vi "Converter_1.0.2_to_1.0.3.vi"() -> ()   [LabVIEW 2014]
uses:
  <vilib>/Utility/xml.llb/Read From XML File(string).vi
panel:
  out "Datenspeicher 2":T1={"Fahrzeugdaten"="", "date/time string"="", "Rolle [Inkr/U]"=0, "Rollenumfang [m]"=0.0, "Rollenträgheit [kgm²]"=0.0, "Zündung [Imp/U]"=0, "Getriebe [1:]"=0.0, "Reifenumfang [m] "=0.0, "element"=0.0, "Gl. Mittelwert"=0, "Differenzenquotient"=0, "Polynom"=0, "element"=0.0, "element"=0.0, "Lufttemperatur [°C]"=0.0, "Luftfeuchtigkeit [%]"=0.0, "Luftdruck [mbar]"=0.0, [], [], "Best Polynomial Fit"=[], [], "Übersetzung ermitteln aus"=0, "[s]"=0.0, "nmin [1/min]"=0.0, "nmax [1/min]"=0.0, "n vom Gas [1/min]"=0.0, [], [], "Boolesch"=FALSE, "Serielle Schnittstelle"="COM4"}
  out "Datenspeicher":T2={"Fahrzeugdaten"="", "date/time string"="", "Rolle [Inkr/U]"=0, "Rollenumfang [m]"=0.0, "Rollenträgheit [kgm²]"=0.0, "Zündung [Imp/U]"=0.0, "Getriebe [1:]"=0.0, "Reifenumfang [m] "=0.0, "element"=0.0, "Gl. Mittelwert"=0, "Differenzenquotient"=0, "Polynom"=0, "element"=0.0, "element"=0.0, "Lufttemperatur [°C]"=0.0, "Luftfeuchtigkeit [%]"=0.0, "Luftdruck [mbar]"=0.0, [], [], "Best Polynomial Fit"=[], [], "Übersetzung ermitteln aus"=0, "[s]"=0.0, "nmin [1/min]"=0.0, "nmax [1/min]"=0.0, "n vom Gas [1/min]"=0.0, [], [], "Boolesch"=FALSE, "Serielle Schnittstelle"="COM4", "nKuWe/nRolle"=10.0}
  # "WildBugChilGru XML Converter"
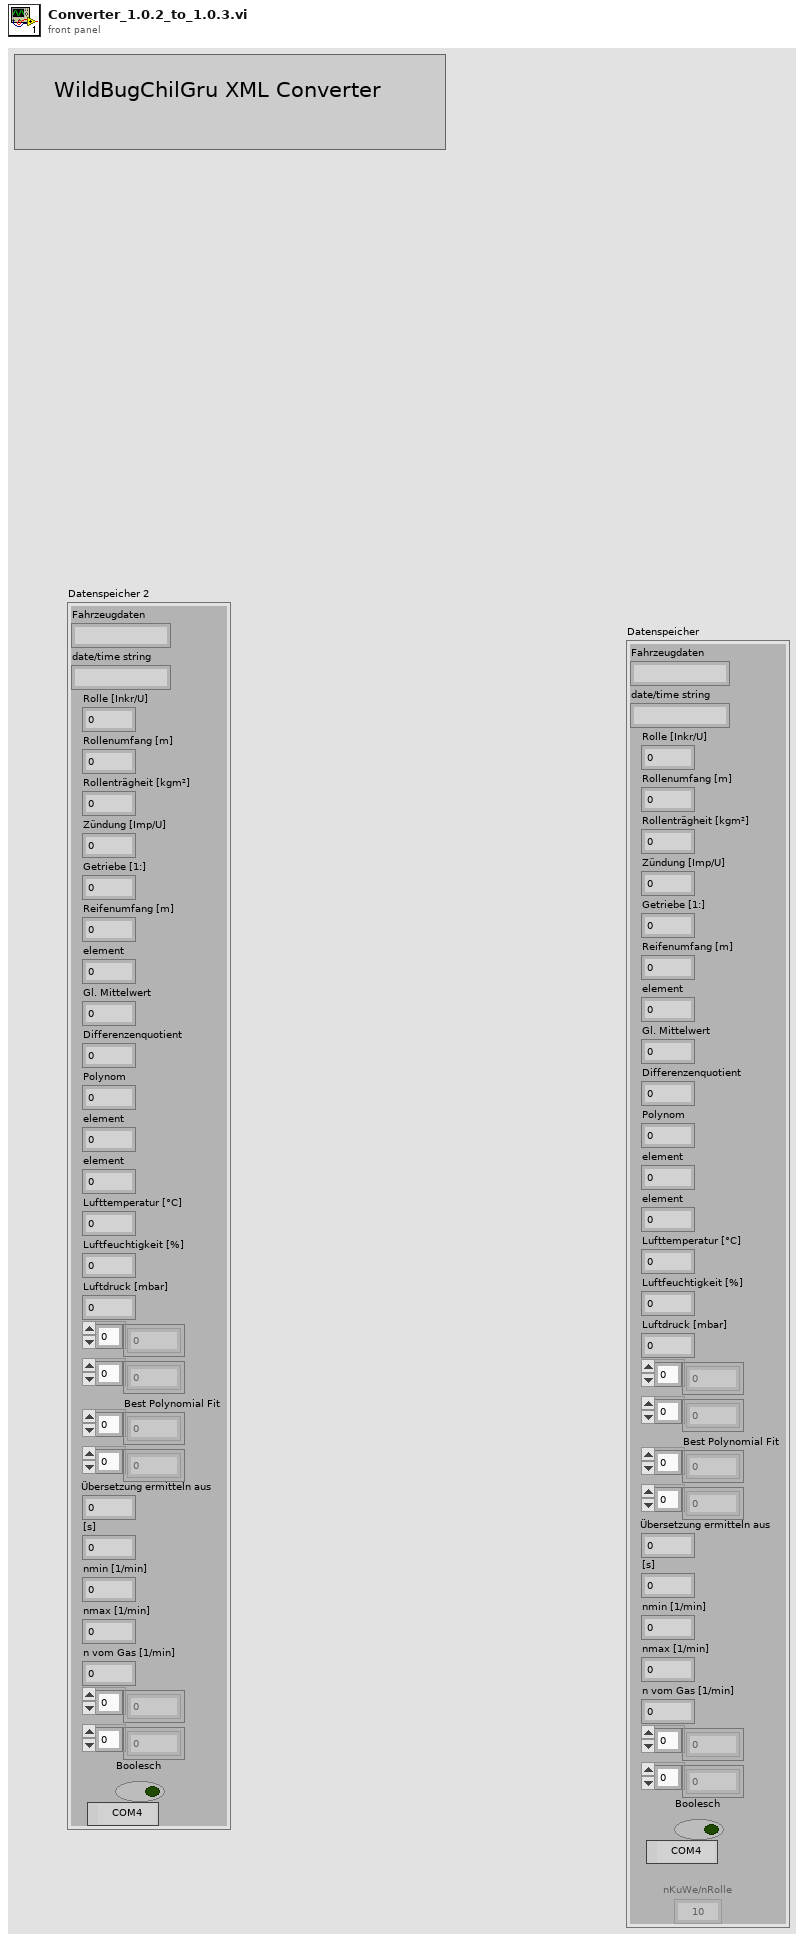
[diagram p1: front panel]
types:
  T1 = cluster{"Fahrzeugdaten":string, "date/time string":string, "Rolle [Inkr/U]":u16, "Rollenumfang [m]":dbl, "Rollenträgheit [kgm²]":dbl, "Zündung [Imp/U]":u8, "Getriebe [1:]":dbl, "Reifenumfang [m] ":dbl, "element":dbl, "Gl. Mittelwert":u8, "Differenzenquotient":u8, "Polynom":u8, "element":dbl, "element":dbl, "Lufttemperatur [°C]":dbl, "Luftfeuchtigkeit [%]":dbl, "Luftdruck [mbar]":dbl, dbl[], dbl[], "Best Polynomial Fit":dbl[], dbl[], "Übersetzung ermitteln aus":u8, "[s]":dbl, "nmin [1/min]":dbl, "nmax [1/min]":dbl, "n vom Gas [1/min]":dbl, dbl[], i32[], "Boolesch":bool, "Serielle Schnittstelle":refnum<visa-resource-name>}
  T2 = cluster{"Fahrzeugdaten":string, "date/time string":string, "Rolle [Inkr/U]":u16, "Rollenumfang [m]":dbl, "Rollenträgheit [kgm²]":dbl, "Zündung [Imp/U]":dbl, "Getriebe [1:]":dbl, "Reifenumfang [m] ":dbl, "element":dbl, "Gl. Mittelwert":u8, "Differenzenquotient":u8, "Polynom":u8, "element":dbl, "element":dbl, "Lufttemperatur [°C]":dbl, "Luftfeuchtigkeit [%]":dbl, "Luftdruck [mbar]":dbl, dbl[], dbl[], "Best Polynomial Fit":dbl[], dbl[], "Übersetzung ermitteln aus":u8, "[s]":dbl, "nmin [1/min]":dbl, "nmax [1/min]":dbl, "n vom Gas [1/min]":dbl, dbl[], i32[], "Boolesch":bool, "Serielle Schnittstelle":refnum<visa-resource-name>, "nKuWe/nRolle":dbl}
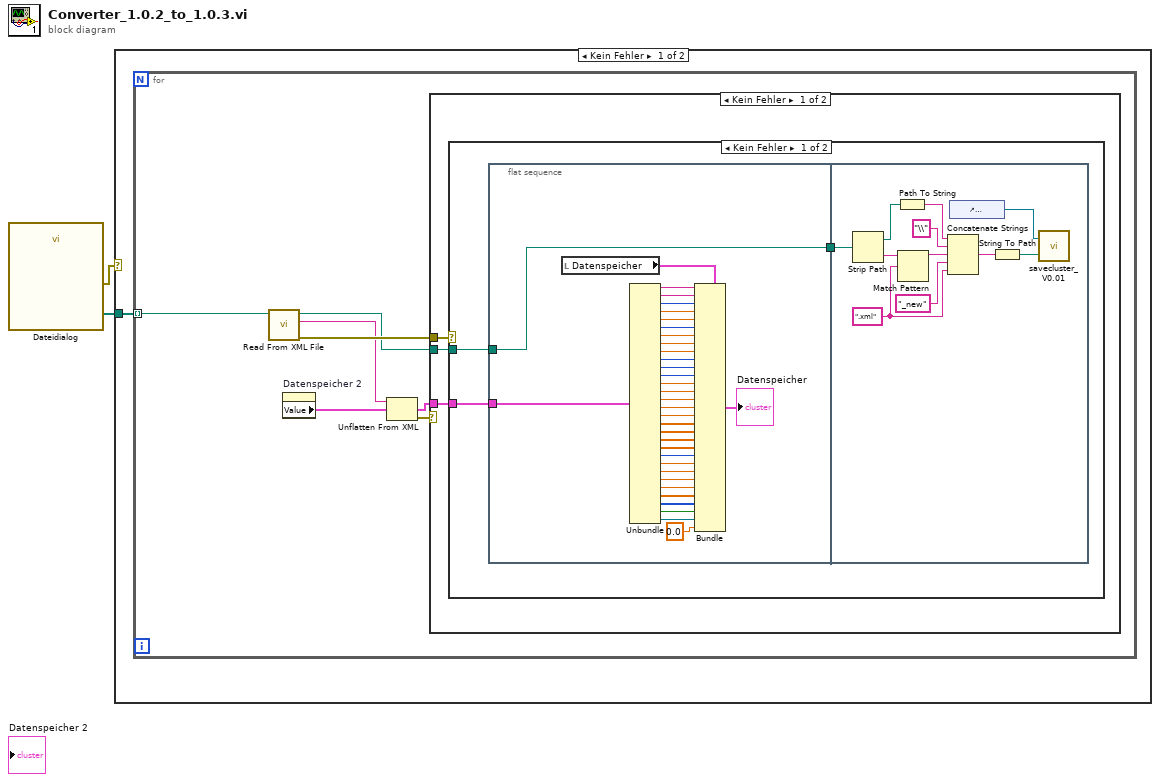
[diagram p0: block diagram]
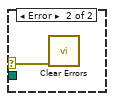
[diagram p2: hidden frame]
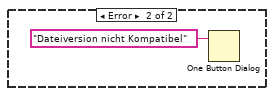
[diagram p3: hidden frame]
diagram:
  n1 = call "Dateidialog"() -> ("selected paths"=w2:path[], "error out"=w1:errorcluster)  [unwired: 12 in, 2 out]
  n2 = case shown="Kein Fehler" w1 {
    tunnel: w2 -> [w3 _]
    frame No Error {
      n3 = for {
        tunnel: w3 -> [w8] mode=indexing
        n4 = call-poly <vilib>:"Read From XML File.vi"("XML File Path"=w8) -> ("error out"=w10:errorcluster, "XML Elements"=w7:string, "XML File Path(duplicate)"=w9:path)  [unwired: 8 in]
        n5 = property on="Datenspeicher 2" class="Cluster (strikt)"() -> ("Value"=w6:T1)  [unwired: 2 in, 2 out]
        n6 = Unflatten From XML(xml string=w7, type=w6) -> (value=w5:T1, error out=w4:errorcluster)  [unwired: 1 in]
        n7 = case shown="Kein Fehler" w4 {
          tunnel: w10 -> [w13 _]
          tunnel: w9 -> [w12 _]
          tunnel: w5 -> [w11 _]
          frame No Error {
            n8 = case shown="Kein Fehler" w13 {
              selector: w13 -> [_ w63]
              tunnel: w12 -> [w15 _]
              tunnel: w11 -> [w14 _]
              frame No Error {
                n9 = flat-sequence {
                  tunnel: w14 -> [w17]
                  tunnel: [w18] -> w16
                  tunnel: w15 -> [w18]
                  tunnel: w16 -> [w62]
                  frame #0 {
                    n10 = local read "Datenspeicher"() -> (w50:T2)
                    n11 = Unbundle(w17) -> ("Fahrzeugdaten"=w49:string, "date/time string"=w48:string, "Rolle [Inkr/U]"=w47:u16, "Rollenumfang [m]"=w46:dbl, "Rollenträgheit [kgm²]"=w20:dbl, "Zündung [Imp/U]"=w21:u8, "Getriebe [1:]"=w22:dbl, "Reifenumfang [m]"=w23:dbl, "element"=w24:dbl, "Gl. Mittelwert"=w25:u8, "Differenzenquotient"=w26:u8, "Polynom"=w27:u8, "element"=w28:dbl, "element"=w29:dbl, "Lufttemperatur [°C]"=w30:dbl, "Luftfeuchtigkeit [%]"=w31:dbl, "Luftdruck [mbar]"=w32:dbl, w33:dbl[], w34:dbl[], "Best Polynomial Fit"=w35:dbl[], w36:dbl[], "Übersetzung ermitteln aus"=w37:u8, "[s]"=w38:dbl, "nmin [1/min]"=w39:dbl, "nmax [1/min]"=w40:dbl, "n vom Gas [1/min]"=w41:dbl, w42:dbl[], w43:i32[], "Boolesch"=w44:bool, "Serielle Schnittstelle"=w45:refnum<visa-resource-name>)
                    n12 = Bundle(cluster=w50, "Fahrzeugdaten"=w49, "date/time string"=w48, "Rolle [Inkr/U]"=w47, "Rollenumfang [m]"=w46, "Rollenträgheit [kgm²]"=w20, "Zündung [Imp/U]"=w21, "Getriebe [1:]"=w22, "Reifenumfang [m]"=w23, "element"=w24, "Gl. Mittelwert"=w25, "Differenzenquotient"=w26, "Polynom"=w27, "element"=w28, "element"=w29, "Lufttemperatur [°C]"=w30, "Luftfeuchtigkeit [%]"=w31, "Luftdruck [mbar]"=w32, w33, w34, "Best Polynomial Fit"=w35, w36, "Übersetzung ermitteln aus"=w37, "[s]"=w38, "nmin [1/min]"=w39, "nmax [1/min]"=w40, "n vom Gas [1/min]"=w41, w42, w43, "Boolesch"=w44, "Serielle Schnittstelle"=w45, "nKuWe/nRolle"=0.0) -> (→"Datenspeicher":T2)
                  }
                  frame #1 {
                    w56 = ".xml" ("Regulärer Ausdruck")
                    n13 = Strip Path(path=w62) -> (stripped path=w58:path, name=w61:string)
                    n14 = Path To String(path=w58) -> (string=w54:string)
                    n15 = Match Pattern(string=w61, regular expression=w56) -> (before substring=w53:string)  [unwired: 1 in, 3 out]
                    n16 = Concatenate Strings(w54, "\\", w53, "_new" ("String"), w56) -> (w59:string)
                    n17 = control-ref of="Datenspeicher"() -> (w55:refnum<vi>)
                    n18 = String To Path(string=w59) -> (path=w57:path)
                    n19 = call "savecluster_V0.01.vi"("selected path"=w57, "Datenspeicher 3"=w55) -> ()  [unwired: 1 in]
                  }
                }
              }
              frame Error {
                n20 = call <vilib>:"Clear Errors.vi"("error in (no error)"=w63) -> ()  [unwired: 5 in, 2 out]
              }
            }
          }
          frame Error {
            n21 = One Button Dialog(message="Dateiversion nicht Kompatibel" ("Nachricht")) -> ()  [unwired: 1 in, 1 out]
          }
        }
      }
    }
    frame Error {
    }
  }
